vi "TCP Data read (SubVI).vi"(8 "error in (no error)":errorcluster, 10 "Запись в файл":bool, 11 "TCP Network Connection in":refnum<k5>) -> (0 "error out":errorcluster, 1 "Запись в файл вых":bool, 2 "Read data":string, 3 "TCP Network Connection out":refnum<k5>)   [LabVIEW 2013]
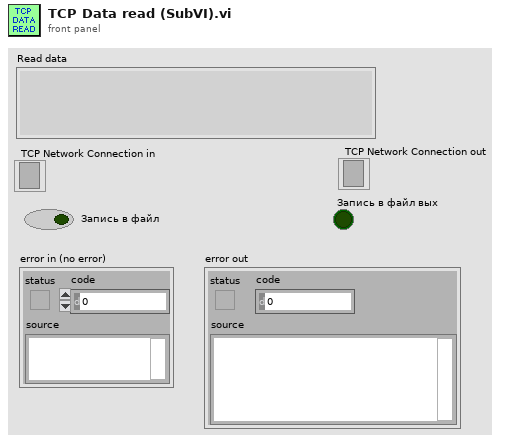
[diagram p1: front panel]
types:
  T1 = enum16{"Standard", "Buffered", "CRLF", "Immediate"}
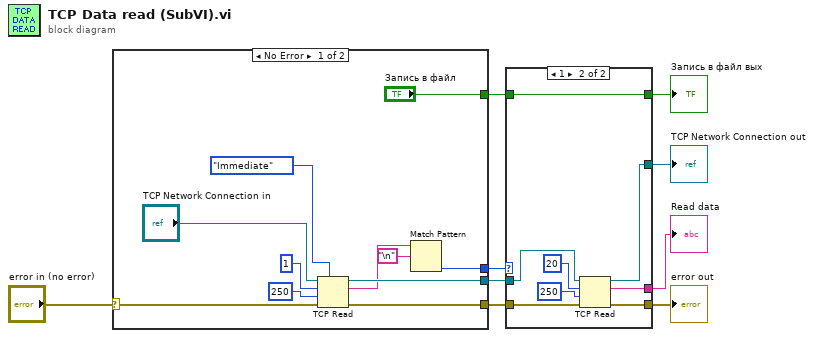
[diagram p0: block diagram]
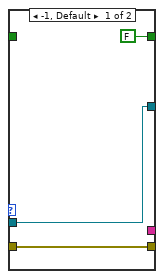
[diagram p2: hidden frame]
diagram:
  n1 = case shown="No Error" "error in (no error)" {
    selector: "error in (no error)" -> [w10 w21]
    tunnel: ["Запись в файл" _] -> w7
    tunnel: [w19 w21] -> w1
    tunnel: [w14 _] -> w6
    tunnel: [w12 _] -> w5
    frame No Error {
      n2 = TCP Read(connection ID="TCP Network Connection in", bytes to read=1, error in (no error)=w10, 7:T1."Immediate" ("mode (standard)"), 9:250 ("timeout ms (25000)")) -> (connection ID out=w12:refnum<k5>, data out=w11:string, error out=w19:errorcluster)
      n3 = Match Pattern(string=w11, regular expression="\n") -> (offset past match=w14:i32)  [unwired: 4 out]
    }
    frame Error {
    }
  }
  n4 = case shown="1" w6 {
    tunnel: [w24 w28] -> w8
    tunnel: [_ w27] -> w9
    tunnel: w5 -> [w22 w32]
    tunnel: w7 -> [_ w26]
    tunnel: w1 -> [w24 w31]
    tunnel: [FALSE ("Запись в файл") w26] -> w4
    tunnel: [w22 w25] -> w3
    frame -1, Default {
    }
    frame 1 {
      n5 = TCP Read(connection ID=w32, bytes to read=20, error in (no error)=w31, 9:250 ("timeout ms (25000)")) -> (connection ID out=w25:refnum<k5>, data out=w27:string, error out=w28:errorcluster)  [unwired: 1 out]
    }
  }
  "Read data" <- w9
  "error out" <- w8
  "Запись в файл вых" <- w4
  "TCP Network Connection out" <- w3
